vi "Configure Data Read.vi"(0 "RedPitaya connection in":refnum<k5>, 2 "Read Units":string(combo), 3 "Data Format":string(combo), 5 "error in":errorcluster, 12 "timeout ms (2000)":i32=2000) -> (14 "RedPitaya connection out":refnum<k5>, 19 "error out":errorcluster)   [LabVIEW 2010, in "RedPitaya.lvlib"]
doc: "Confugures units and format in which the acquired data will be returned."
uses:
  RedPitaya.lvlib
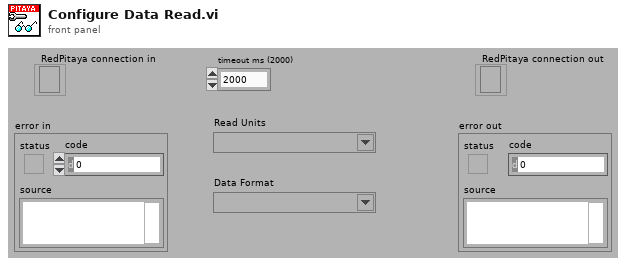
[diagram p1: front panel]
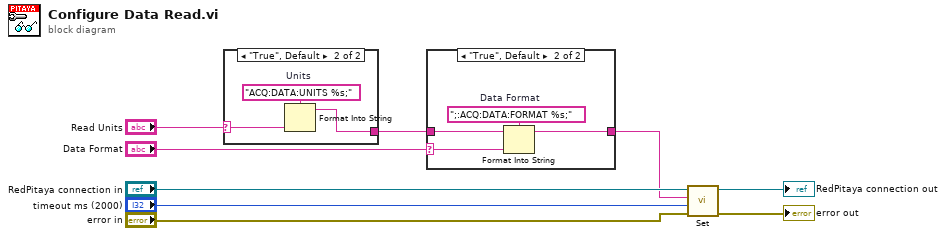
[diagram p0: block diagram]
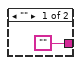
[diagram p3: hidden frame]
diagram:
  n1 = case shown="\"True\", Default" "Read Units" {
    selector: "Read Units" -> [_ w11]
    tunnel: ["" w12] -> w5
    frame "" {
    }
    frame "True", Default {
      w13 = "ACQ:DATA:UNITS %s;"  # Units
      n2 = Format Into String(format string=w13, w11) -> (resulting string=w12:string)  [unwired: 2 in, 1 out]
    }
  }
  n3 = case shown="\"True\", Default" "Data Format" {
    selector: "Data Format" -> [_ w15]
    tunnel: w5 -> [w14 w17]
    tunnel: [w14 w16] -> w2
    frame "" {
    }
    frame "True", Default {
      w18 = ";:ACQ:DATA:FORMAT %s;"  # Data Format
      n4 = Format Into String(format string=w18, initial string=w17, w15) -> (resulting string=w16:string)  [unwired: 1 in, 1 out]
    }
  }
  n5 = call "Set.vi"("error in"="error in", "timeout ms (2000)"="timeout ms (2000)", "SCPI Message"=w2, "RedPitaya connection in"="RedPitaya connection in") -> ("error out"=→"error out":errorcluster, "RedPitaya connection out"=→"RedPitaya connection out":refnum<k5>)  [unwired: 5 in, 1 out]
